vi "Package Measurement.vi"() -> ()   [LabVIEW 2021]
uses:
  _Measurement Packager Utility/Packager Helpers/Queue Driver/controls/Queue Operations.ctl
  <vilib>/Utility/miscctls.llb/LVRowAndColumnTypeDef.ctl
  _Measurement Packager Utility/Packager Helpers/controls/Config File Operations.ctl
  _Measurement Packager Utility/Packager Helpers/controls/Data Holder.ctl
  <vilib>/Utility/miscctls.llb/LVPoint32TypeDef.ctl
  _Measurement Packager Utility/Packager Helpers/controls/Build Spec Details.ctl
  <vilib>/AppBuilder/AB_API_Simple/Get Build Specification Version (path).vi
  _Measurement Packager Utility/Packager Helpers/Queue Driver/Queue Driver.lvlib
  _Measurement Packager Utility/Packager Helpers/Packager Helpers.lvlib
  _Measurement Packager Utility/Packager Helpers/Dictionary/Dictionary.lvlib
  <vilib>/AppBuilder/AB_API_Simple/NI_App_Builder_API.lvlib
panel:
  out "error out":errorcluster
  out "Tab Control":T1(tab)
  in  "Open Directory":bool
  in  "Feed Path":path
  out "Warning":bool=TRUE caption="Feed Path cannot be empty/invalid"
  in  "Next to select":bool
  in  "Build Package":bool
  in  "Project":path caption="LabVIEW Project Path"
  in  "Feed":T2(radio)
  in  "Back 1":bool
  in  "Populate Package":bool
  in  "Select All":bool
  out "Measurement List":i32(listbox)=-1 caption="Select the Measurements to build the package"
  out "Selection warning":string="Selected Project doesn't have EXE build spec"
  out "Maintainer Warning":string
  in  "Settings Page":enum32{"Page 1", "Page 2"}(tab)
  in  "Maintainer Email ID":string="sabthagiri@ni.com"
  in  "Architecture":string(combo)="1"
  in  "Maintainer":string="NI"
  in  "Back 2":bool
  in  "Start Build":bool
  in  "Package List":i32[](listbox) caption="Edit the Package Name and Version"
  in  "Settings":bool
  in  "Progres Bar":i32(slide)=9 caption="Creating Distribution..." scale=0.0..100.0
  in  "Start Next":bool
  in  "Log":bool[](array[boolean])=[TRUE, TRUE]
  in  "Build Status":i32(listbox)=-1
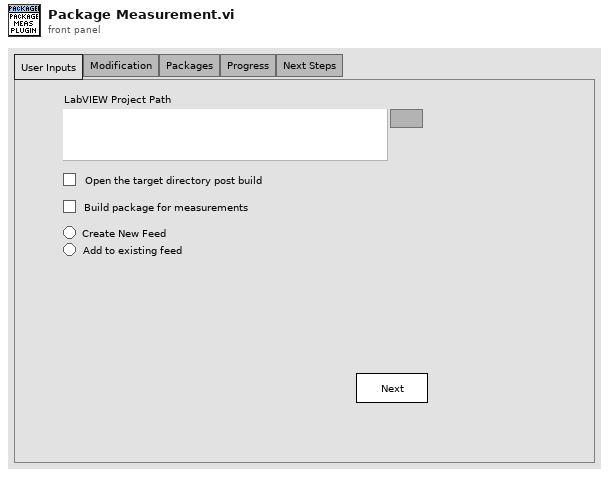
[diagram p1: front panel]
types:
  T1 = enum32{"User Inputs", "Modification", "Packages", "Progress", "Next Steps"}
  T2 = enum32{"No Selection", "CreateFeed", "AddtoFeed"}
  T3 = typedef "LVRowAndColumnTypeDef.ctl" = cluster{"Row":i32, "Column":i32}
  T4 = typedef "Queue Driver.lvlib/Queue Operations.ctl" = enum16{"Create Q", "Enqueue", "Enqueue N", "Dequeue", "Flush", "Release"}
  T5 = enum8{"Enabled", "Disabled", "Disabled and Grayed Out"}
  T6 = typedef "Packager Helpers.lvlib/Config File Operations.ctl" = enum16{"Read", "Write"}
  T7 = typedef "Packager Helpers.lvlib/Data Holder.ctl" = cluster{"Next Clicked?":bool, "MosueDown Coords":T8, "Build Spec":T9[], "No of Meas":i32, "No. of Selected Meas":i32, "Selected Meas":T9[], "Package Details":string[][], "Build Packge?":bool, "Packages Path":path, "Feed":enum32{"No Selection", "CreateFeed", "AddtoFeed"}, "Feed Path":path, "Valid Inputs?":bool, "Feed Old":enum32{"No Selection", "CreateFeed", "AddtoFeed"}, "Status":string[], "Open Directory?":bool}
  T8 = typedef "LVPoint32TypeDef.ctl" = cluster{"Horizontal":i32, "Vertical":i32}
  T9 = typedef "Packager Helpers.lvlib/Build Spec Details.ctl" = cluster{"EXE Name":string, "Target path":path, "Has PPL?":bool, "PPL Name":string}
  T10 = typedef "NI_App_Builder_API.lvlib/Build Specification Version.ctl" = cluster{"Major":u16, "Minor":u16, "Fix":u16, "Build":u16}
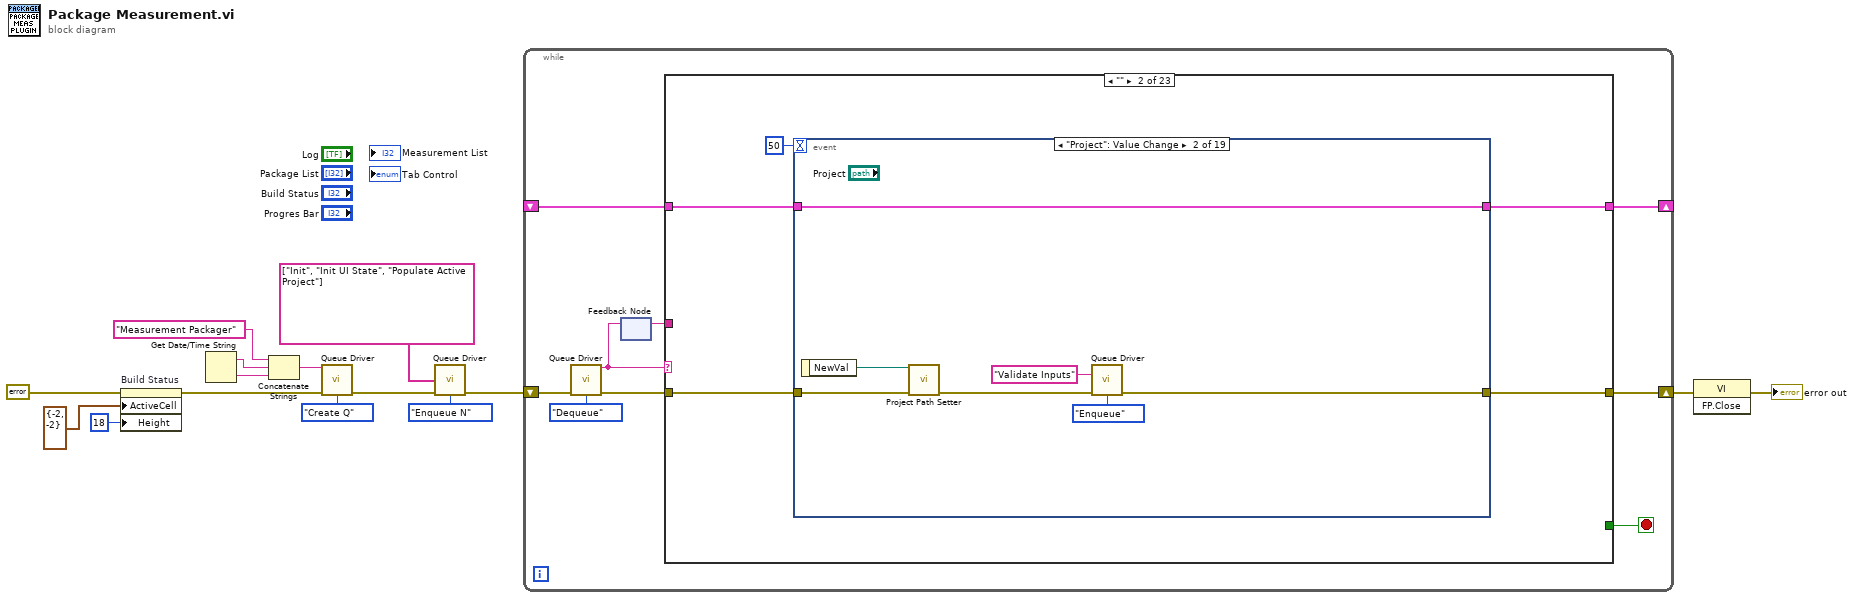
[diagram p0: block diagram]
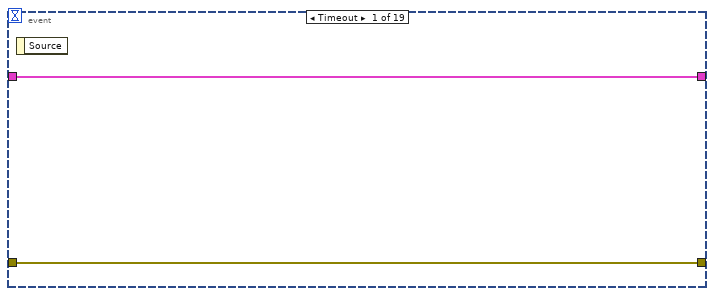
[diagram p3: hidden frame]
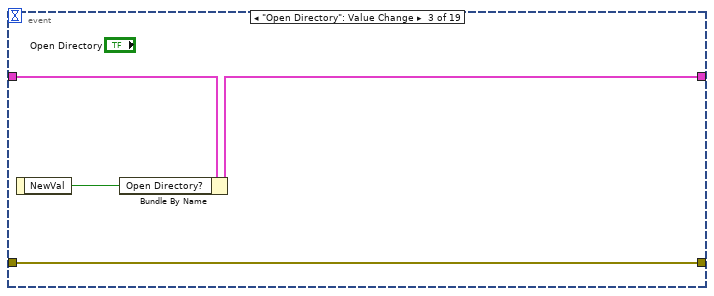
[diagram p4: hidden frame]
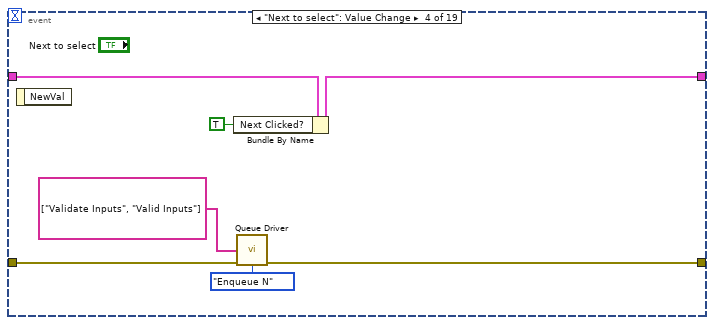
[diagram p5: hidden frame]
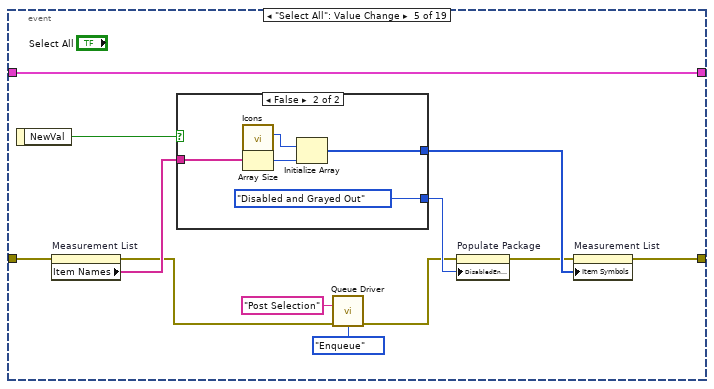
[diagram p6: hidden frame]
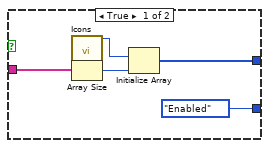
[diagram p7: hidden frame]
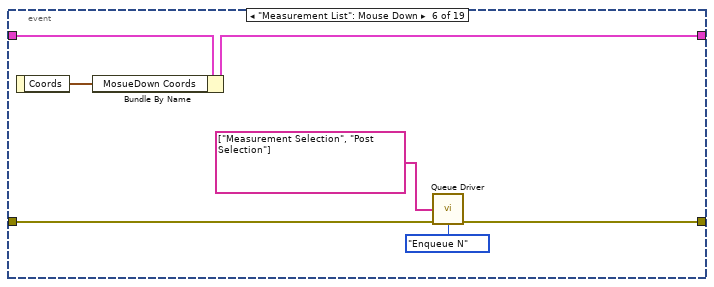
[diagram p8: hidden frame]
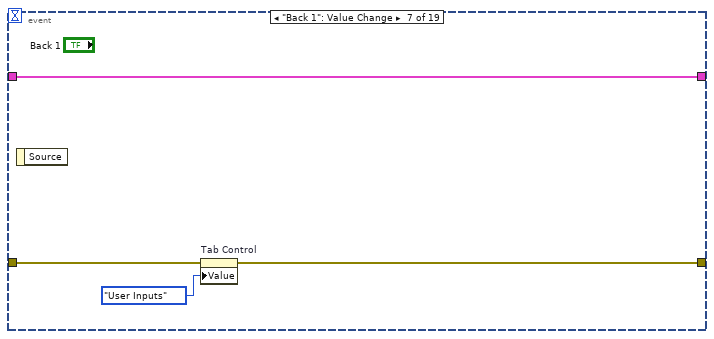
[diagram p9: hidden frame]
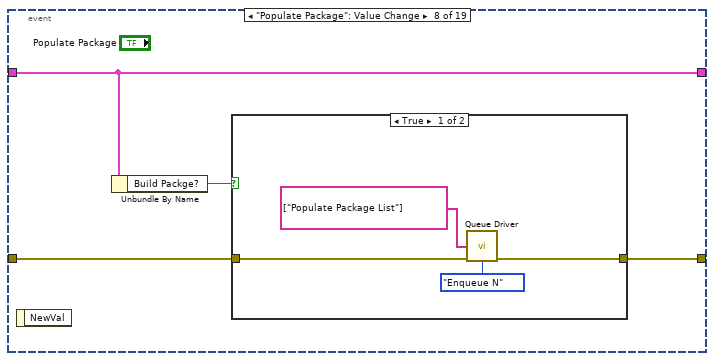
[diagram p10: hidden frame]
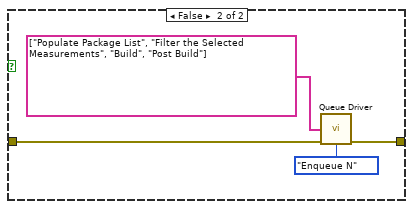
[diagram p11: hidden frame]
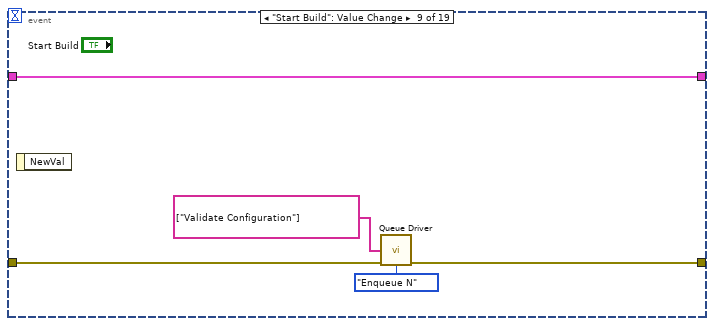
[diagram p12: hidden frame]
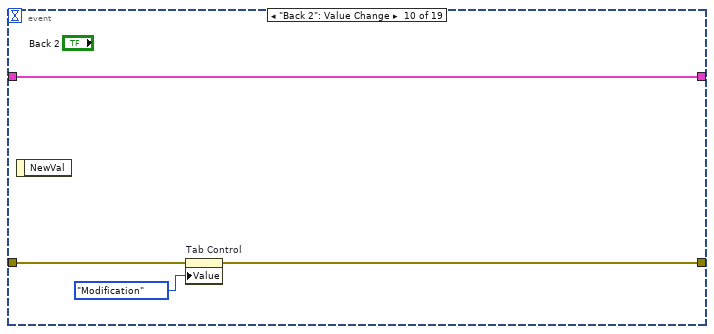
[diagram p13: hidden frame]
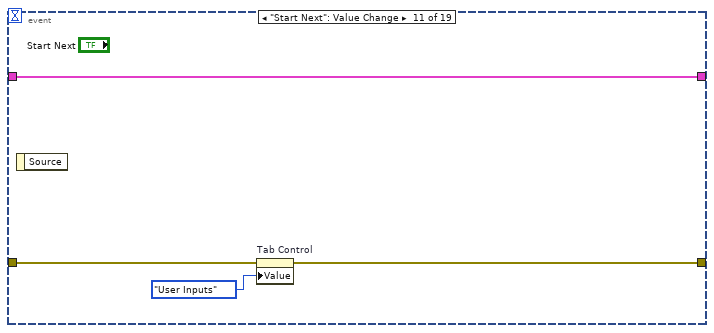
[diagram p14: hidden frame]
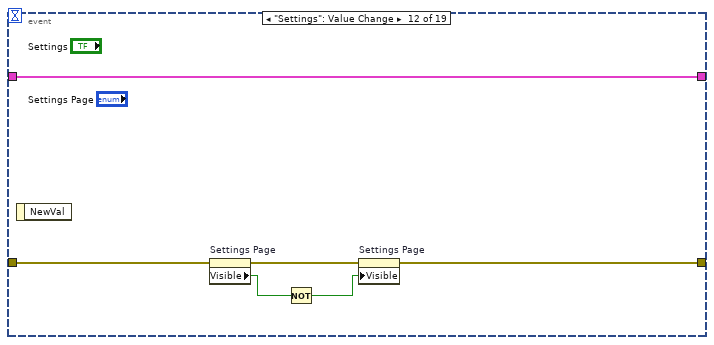
[diagram p15: hidden frame]
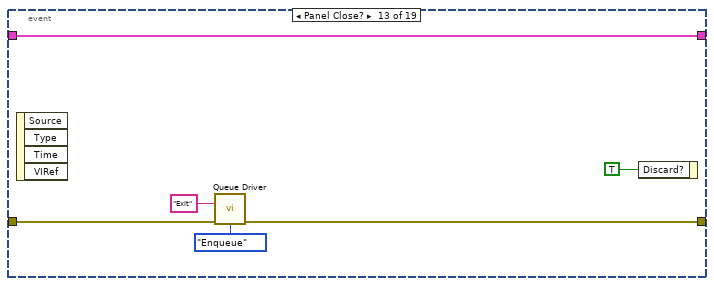
[diagram p16: hidden frame]
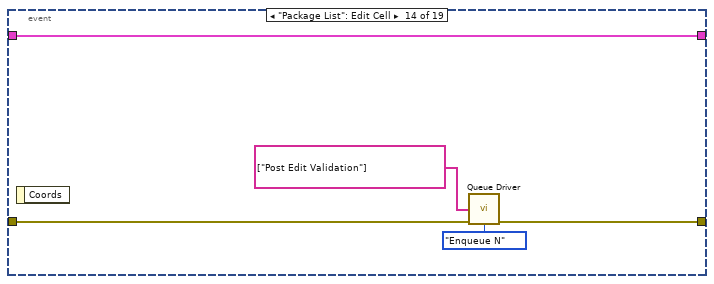
[diagram p17: hidden frame]
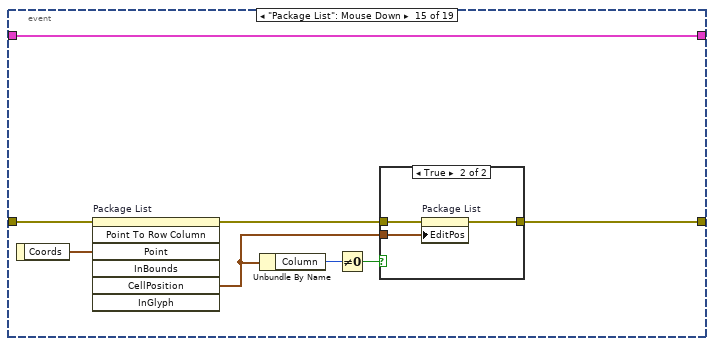
[diagram p18: hidden frame]
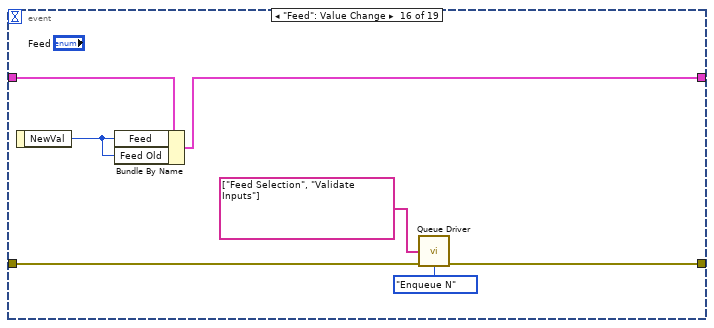
[diagram p20: hidden frame]
diagram:
  n1 = property on="Build Status" class="MCListbox (strict)"(error in=errorcluster {"status"=FALSE, "code"=0, "source"=""} ("error in (no error)"), "ActiveCell"=T3 {"Row"=-2, "Column"=-2} ("Active Cell:Active Cell"), "Height"=u32 18 ("Active Cell:Cell Size:Height")) -> (error out=w8:errorcluster)  [unwired: 1 in, 1 out]
  n2 = Get Date/Time String() -> (date string=w2:string, time string=w10:string)  [unwired: 3 in]
  n3 = Concatenate Strings("Measurement Packager" ("string"), w2, w10) -> (w9:string)
  n4 = call "Queue Driver.vi"("Name"=w9, "error in (no error)"=w8, "Queue Operations"=Queue_Operations."Create Q" ("Q Operations")) -> ("error out"=w13:errorcluster)  [unwired: 11 in, 1 out]
  n5 = call "Queue Driver.vi"("States[]"=string[] ["Init", "Init UI State", "Populate Active Project"], "error in (no error)"=w13, "Queue Operations"=Queue_Operations."Enqueue N" ("Q Operations")) -> ("error out"=w15:errorcluster)  [unwired: 11 in, 1 out]
  n6 = while {
    shift-right: [w17] -> w4
    shift-left: w15 -> [w24]
    shift-right: [w21] -> _
    shift-left: _ -> [w20]
    stop <- w18 stop-if-true
    n7 = call "Queue Driver.vi"("error in (no error)"=w24, "Queue Operations"=Queue_Operations."Dequeue" ("Q Operations")) -> ("Dequeued State"=w16:string, "error out"=w22:errorcluster)  [unwired: 12 in]
    n8 = feedback #1() -> (w19:string)  [unwired: 1 in]
    n9 = feedback-in #1(w16) -> ()
    n10 = case shown="\"\"" w16 {
      tunnel: w22 -> [w25 w31 w170 w182 w196 w217 w229 w283 w300 w320 w335 w358 w377 w391 w397 w418 w454 w458 w472 w486 w502 w515 w520]
      tunnel: [w25 w27 w168 w173 w190 w216 w233 w282 w303 w319 w332 w350 w378 w390 w394 w412 w453 w456 w469 w481 w500 w511 w522] -> w17
      tunnel: [w26 w30 w171 w186 w204 w218 w232 w281 w305 w321 w337 w360 w385 w393 w404 w421 w455 w459 w465 w499 w504 w518 w523] -> w21
      tunnel: w20 -> [w26 w29 _ w186 w205 w218 w231 w281 w297 w321 w337 w360 w386 w393 w404 w419 w455 w461 w465 w495 w504 w518 w523]
      tunnel: w19 -> [_ _ _ _ _ _ _ _ _ _ _ _ _ _ _ _ _ _ _ _ _ _ _]
      tunnel: [_ _ _ _ _ _ _ _ _ _ _ _ _ _ _ _ _ _ _ _ _ _ TRUE] -> w18
      frame Default {
      }
      frame "" {
        n11 = event shown="[1] \"Project\": Value Change" {
          selector: _ -> [_ _ _ _ _ _ _ _ _ _ _ _ _ _ _ _ _ _ _]
          dyn-events: _ -> [_ _ _ _ _ _ _ _ _ _ _ _ _ _ _ _ _ _ _]
          timeout: 50 -> [_ _ _ _ _ _ _ _ _ _ _ _ _ _ _ _ _ _ _]
          tunnel: [w32 w34 w41 w45 w52 w75 w81 w85 w97 w104 w108 w112 w116 w122 w128 w139 w147 w153 w160] -> w27
          tunnel: w31 -> [w32 w36 w41 w46 w56 w74 w82 w86 w98 w105 w109 w113 w117 w123 w127 w140 w146 w154 w161]
          tunnel: [w33 w39 w43 w49 w63 w79 w84 w88 w101 w103 w107 w110 w120 w126 w134 w144 w151 w159 w165] -> w30
          tunnel: w29 -> [w33 w39 w44 w50 w63 w80 w84 w88 w101 w103 w107 w110 w120 w126 w134 w145 w152 w159 w166]
          event Timeout {
            n12 = event-data() -> ()  [unwired: 1 in, 1 out]
          }
          event "Project": Value Change {
            n13 = event-data() -> ("NewVal"=w38:path)  [unwired: 1 in]
            n14 = call "Project Path Setter.vi"("ProjectPath In"=w38, "error in (no error)"=w36) -> ("error out"=w35:errorcluster)  [unwired: 13 in]
            n15 = call "Queue Driver.vi"("State"="Validate Inputs", "error in (no error)"=w35, "Queue Operations"=Queue_Operations."Enqueue" ("Q Operations")) -> ("error out"=w34:errorcluster)  [unwired: 11 in, 1 out]
          }
          event "Open Directory": Value Change {
            n16 = event-data() -> ("NewVal"=w42:bool)  [unwired: 1 in]
            n17 = Bundle By Name(cluster=w44, "Open Directory?"=w42) -> (w43:T7)
          }
          event "Next to select": Value Change {
            n18 = event-data() -> ()  [unwired: 1 in, 1 out]
            n19 = Bundle By Name(cluster=w50, "Next Clicked?"=TRUE) -> (w49:T7)
            n20 = call "Queue Driver.vi"("States[]"=string[] ["Validate Inputs", "Valid Inputs"], "error in (no error)"=w46, "Queue Operations"=Queue_Operations."Enqueue N" ("Q Operations")) -> ("error out"=w45:errorcluster)  [unwired: 11 in, 1 out]
          }
          event "Select All": Value Change {
            n21 = event-data() -> ("NewVal"=w58:bool)  [unwired: 1 in]
            n22 = property on="Measurement List" class="LstBox (strict)"(error in=w56) -> (error out=w55:errorcluster, "Item Names"=w62:string[])  [unwired: 1 in, 1 out]
            n23 = case shown="False" w58 {
              tunnel: w62 -> [w67 w72]
              tunnel: [w66 w71] -> w61
              tunnel: [T5."Enabled" ("Disabled") T5."Disabled and Grayed Out" ("Disabled")] -> w60
              frame True {
                n24 = call "Icons.vi"() -> ("Selected"=w64:i32)  [unwired: 14 in, 1 out]
                n25 = Array Size(array=w67) -> (size(s)=w68:i32)
                n26 = Initialize Array(w64, w68) -> (w66:i32[])
              }
              frame False {
                n27 = call "Icons.vi"() -> ("Non Selected"=w70:i32)  [unwired: 14 in, 1 out]
                n28 = Array Size(array=w72) -> (size(s)=w73:i32)
                n29 = Initialize Array(w70, w73) -> (w71:i32[])
              }
            }
            n30 = call "Queue Driver.vi"("State"="Post Selection", "error in (no error)"=w55, "Queue Operations"=Queue_Operations."Enqueue" ("Q Operations")) -> ("error out"=w54:errorcluster)  [unwired: 11 in, 1 out]
            n31 = property on="Populate Package" class="Bool"(error in=w54, "DisabledEnum"=w60) -> (error out=w53:errorcluster)  [unwired: 1 in, 1 out]
            n32 = property on="Measurement List" class="LstBox (strict)"(error in=w53, "Item Symbols"=w61) -> (error out=w52:errorcluster)  [unwired: 1 in, 1 out]
          }
          event "Measurement List": Mouse Down {
            n33 = event-data() -> ("Coords"=w77:T8)  [unwired: 1 in]
            n34 = Bundle By Name(cluster=w80, "MosueDown Coords"=w77) -> (w79:T7)
            n35 = call "Queue Driver.vi"("States[]"=string[] ["Measurement Selection", "Post Selection"], "error in (no error)"=w74, "Queue Operations"=Queue_Operations."Enqueue N" ("Q Operations")) -> ("error out"=w75:errorcluster)  [unwired: 11 in, 1 out]
          }
          event "Back 1": Value Change {
            n36 = event-data() -> ()  [unwired: 1 in, 1 out]
            n37 = property on="Tab Control" class="TabCtl (strict)"(error in=w82, "Value"=T1."User Inputs" ("Tab Control")) -> (error out=w81:errorcluster)  [unwired: 1 in, 1 out]
          }
          event "Populate Package": Value Change {
            n38 = event-data() -> ()  [unwired: 1 in, 1 out]
            n39 = Unbundle By Name(w88) -> ("Build Packge?"=w87:bool)
            n40 = case shown="True" w87 {
              tunnel: w86 -> [w90 w94]
              tunnel: [w89 w93] -> w85
              frame True {
                n41 = call "Queue Driver.vi"("States[]"=string[] ["Populate Package List"], "error in (no error)"=w90, "Queue Operations"=Queue_Operations."Enqueue N" ("Q Operations")) -> ("error out"=w89:errorcluster)  [unwired: 11 in, 1 out]
              }
              frame False {
                n42 = call "Queue Driver.vi"("States[]"=string[] ["Populate Package List", "Filter the Selected Measurements", "Build", "Post Build"], "error in (no error)"=w94, "Queue Operations"=Queue_Operations."Enqueue N" ("Q Operations")) -> ("error out"=w93:errorcluster)  [unwired: 11 in, 1 out]
              }
            }
          }
          event "Start Build": Value Change {
            n43 = event-data() -> ()  [unwired: 1 in, 1 out]
            n44 = call "Queue Driver.vi"("States[]"=string[] ["Validate Configuration"], "error in (no error)"=w98, "Queue Operations"=Queue_Operations."Enqueue N" ("Q Operations")) -> ("error out"=w97:errorcluster)  [unwired: 11 in, 1 out]
          }
          event "Back 2": Value Change {
            n45 = event-data() -> ()  [unwired: 1 in, 1 out]
            n46 = property on="Tab Control" class="TabCtl (strict)"(error in=w105, "Value"=T1."Modification" ("Tab Control")) -> (error out=w104:errorcluster)  [unwired: 1 in, 1 out]
          }
          event "Start Next": Value Change {
            n47 = event-data() -> ()  [unwired: 1 in, 1 out]
            n48 = property on="Tab Control" class="TabCtl (strict)"(error in=w109, "Value"=T1."User Inputs" ("Tab Control")) -> (error out=w108:errorcluster)  [unwired: 1 in, 1 out]
          }
          event "Settings": Value Change {
            n49 = event-data() -> ()  [unwired: 1 in, 1 out]
            n50 = property on="Settings Page" class="TabCtl (strict)"(error in=w113) -> (error out=w111:errorcluster, "Visible"=w115:bool)  [unwired: 1 in, 1 out]
            n51 = Not(x=w115) -> (.not. x?=w114:bool)
            n52 = property on="Settings Page" class="TabCtl (strict)"(error in=w111, "Visible"=w114) -> (error out=w112:errorcluster)  [unwired: 1 in, 1 out]
          }
          event Panel Close? {
            n53 = event-data() -> ()  [unwired: 1 in, 4 out]
            n54 = call "Queue Driver.vi"("State"="Exit", "error in (no error)"=w117, "Queue Operations"=Queue_Operations."Enqueue" ("Q Operations")) -> ("error out"=w116:errorcluster)  [unwired: 11 in, 1 out]
            n55 = event-data("Discard?"=TRUE) -> ()  [unwired: 1 in, 1 out]
          }
          event "Package List": Edit Cell {
            n56 = event-data() -> ()  [unwired: 1 in, 1 out]
            n57 = call "Queue Driver.vi"("States[]"=string[] ["Post Edit Validation"], "error in (no error)"=w123, "Queue Operations"=Queue_Operations."Enqueue N" ("Q Operations")) -> ("error out"=w122:errorcluster)  [unwired: 11 in, 1 out]
          }
          event "Package List": Mouse Down {
            n58 = event-data() -> ("Coords"=w133:T8)  [unwired: 1 in]
            n59 = invoke on="Package List" class="MCListbox (strict)" method="Point To Row Column"(error in=w127, "Point"=w133) -> (error out=w129:errorcluster, "CellPosition"=w130:T3)  [unwired: 5 in, 5 out]
            n60 = Unbundle By Name(w130) -> ("Column"=w132:i32)
            n61 = Not Equal To 0?(x=w132) -> (x != 0?=w131:bool)
            n62 = case shown="True" w131 {
              tunnel: w130 -> [_ w138]
              tunnel: w129 -> [w135 w137]
              tunnel: [w135 w136] -> w128
              frame False {
              }
              frame True {
                n63 = property on="Package List" class="MCListbox (strict)"(error in=w137, "EditPos"=w138) -> (error out=w136:errorcluster)  [unwired: 1 in, 1 out]
              }
            }
          }
          event "Feed": Value Change {
            n64 = event-data() -> ("NewVal"=w141:T2)  [unwired: 1 in]
            n65 = Bundle By Name(cluster=w145, "Feed"=w141, "Feed Old"=w141) -> (w144:T7)
            n66 = call "Queue Driver.vi"("States[]"=string[] ["Feed Selection", "Validate Inputs"], "error in (no error)"=w140, "Queue Operations"=Queue_Operations."Enqueue N" ("Q Operations")) -> ("error out"=w139:errorcluster)  [unwired: 11 in, 1 out]
          }
          event "Build Package": Value Change {
            n67 = event-data() -> ("NewVal"=w148:bool)  [unwired: 1 in]
            n68 = Bundle By Name(cluster=w152, "Build Packge?"=w148) -> (w151:T7)
            n69 = call "Queue Driver.vi"("States[]"=string[] ["Build Package Value Change", "Validate Inputs"], "error in (no error)"=w146, "Queue Operations"=Queue_Operations."Enqueue N" ("Q Operations")) -> ("error out"=w147:errorcluster)  [unwired: 11 in, 1 out]
          }
          event "Architecture", "Maintainer", "Maintainer Email ID": Value Change {
            n70 = event-data() -> ()  [unwired: 1 in, 1 out]
            n71 = call "Read or Write Configurations.vi"("Architecture"="Architecture", "Maintainer"="Maintainer", "Email"="Maintainer Email ID", "error in (no error)"=w154, "Operation"=Config_File_Operations."Write") -> ("error out"=w153:errorcluster)  [unwired: 7 in, 3 out]
          }
          event "Feed Path": Value Change {
            n72 = event-data() -> ("NewVal"=w162:path)  [unwired: 1 in]
            n73 = Bundle By Name(cluster=w166, "Feed Path"=w162) -> (w165:T7)
            n74 = call "Queue Driver.vi"("States[]"=string[] ["Validate Inputs"], "error in (no error)"=w161, "Queue Operations"=Queue_Operations."Enqueue N" ("Q Operations")) -> ("error out"=w160:errorcluster)  [unwired: 11 in, 1 out]
          }
        }
      }
      frame "Init" {
        w167 = TRUE ("Open Directory?")
        n75 = invoke class="VI" method="Default Vals.Reinit All"(error in=w170) -> (error out=w169:errorcluster)  [unwired: 2 in, 2 out]
        n76 = property on="Open Directory" class="Bool (strict)"(error in=w169, "Value"=w167) -> (error out=w168:errorcluster)  [unwired: 1 in, 1 out]
        n77 = Bundle By Name(cluster=T7 {"Next Clicked?"=TRUE, "MosueDown Coords"={"Horizontal"=0, "Vertical"=0}, "Build Spec"=[], "No of Meas"=0, "No. of Selected Meas"=0, "Selected Meas"=[], "Package Details"=[], "Build Packge?"=FALSE, "Packages Path"=path "", "Feed"=enum."No Selection", "Feed Path"=path "", "Valid Inputs?"=FALSE, "Feed Old"=enum."No Selection", "Status"=[], "Open Directory?"=FALSE}, "Open Directory?"=w167) -> (w171:T7)
      }
      frame "Init UI State" {
        w183 = u32 16448250 ("Selection Color")
        w184 = FALSE ("Visible")
        n78 = property on="Tab Control" class="TabCtl (strict)"(error in=w182, "Value"=T1."User Inputs" ("Tab Control")) -> (error out=w181:errorcluster)  [unwired: 1 in, 1 out]
        n79 = property on="Settings Page" class="TabCtl (strict)"(error in=w181, "Visible"=w184) -> (error out=w180:errorcluster)  [unwired: 1 in, 1 out]
        n80 = property on="Warning" class="Bool"(error in=w180, "Visible"=w184) -> (error out=w179:errorcluster)  [unwired: 1 in, 1 out]
        n81 = property on="Selection warning" class="Str"(error in=w179, "Visible"=w184) -> (error out=w178:errorcluster)  [unwired: 1 in, 1 out]
        n82 = property on="Feed Path" class="Path"(error in=w178, "Visible"=w184) -> (error out=w177:errorcluster)  [unwired: 1 in, 1 out]
        n83 = property on="Settings" class="Bool"(error in=w177, "Visible"=w184) -> (error out=w176:errorcluster)  [unwired: 1 in, 1 out]
        n84 = property on="Measurement List" class="LstBox (strict)"(error in=w176, "SelColor"=w183) -> (error out=w175:errorcluster)  [unwired: 1 in, 1 out]
        n85 = property on="Package List" class="MCListbox (strict)"(error in=w175, "SelColor"=w183) -> (error out=w174:errorcluster)  [unwired: 1 in, 1 out]
        n86 = property on="Build Status" class="MCListbox (strict)"(error in=w174, "SelColor"=w183) -> (error out=w173:errorcluster)  [unwired: 1 in, 1 out]
        "Selection warning" <- "Atleast one measurement should be selected" ("Selection warning")
        "Maintainer Warning" <- "Maintainer and Email ID cannot be empty" ("Maintainer Warning")
        "Warning" <- TRUE ("Warning")
      }
      frame "Populate Active Project" {
        # "Get the active labview project"
        n87 = call "Get Active ProjectPath.vi"("error in (no error)"=w196) -> ("Project Path"=w197:path, "error out"=w195:errorcluster)  [unwired: 13 in]
        n88 = property on="Project" class="Path"(error in=w195, "Value"=w197) -> (error out=w194:errorcluster)  [unwired: 1 in, 1 out]
        n89 = call "Project Path Setter.vi"("ProjectPath In"=w197, "error in (no error)"=w194) -> ("error out"=w193:errorcluster)  [unwired: 13 in]
        n90 = Empty String/Path?(string/path=w197) -> (empty?=w200:bool)
        n91 = Not A Number/Path/Refnum?(number/path/refnum=w197) -> (NaN/Path/Refnum?=w199:bool)
        n92 = Or(x=w199, y=w200) -> (x .or. y?=w198:bool)
        n93 = case "Not a valid path?" shown="False" w198 {
          tunnel: w205 -> [w210 w215]
          tunnel: [w209 w214] -> w204
          tunnel: [w207 w213] -> w203
          tunnel: [T5."Disabled and Grayed Out" ("Disabled") T5."Enabled" ("Disabled")] -> w201
          frame True {
            w207 = T2."No Selection" ("Feed")
            n94 = Bundle By Name(cluster=w210, "Build Packge?"=FALSE, "Feed"=w207) -> (w209:T7)
          }
          frame False {
            w213 = T2."CreateFeed" ("Feed")
            n95 = Bundle By Name(cluster=w215, "Build Packge?"=TRUE, "Feed"=w213) -> (w214:T7)
          }
        }
        n96 = Not(x=w198) -> (.not. x?=w202:bool)
        n97 = property on="Build Package" class="Bool (strict)"(error in=w193, "Value"=w202) -> (error out=w192:errorcluster)  [unwired: 1 in, 1 out]
        n98 = property on="Feed" class="RadioBtnsControl (strict)"(error in=w192, "DisabledEnum"=w201) -> (error out=w191:errorcluster)  [unwired: 1 in, 1 out]
        n99 = property on="Feed" class="RadioBtnsControl (strict)"(error in=w191, "Value"=w203) -> (error out=w190:errorcluster)  [unwired: 1 in, 1 out]
      }
      frame "Populate Config" {
        # "Disabling it because the config will not be populated in UI"
        # "Populate Config Data"
        n100 = disable-structure shown="Disabled" {
          disable-tunnel: w217 -> [w223 w228]
          disable-tunnel: [w219 w228] -> w216
          frame Disabled {
            n101 = call "Read or Write Configurations.vi"("error in (no error)"=w223, "Operation"=Config_File_Operations."Read") -> ("Architecture Out"=w226:string, "Maintainer Out"=w225:string, "Email Out"=w224:string, "error out"=w222:errorcluster)  [unwired: 10 in]
            n102 = property on="Maintainer Email ID" class="Str"(error in=w222, "Value"=w224) -> (error out=w221:errorcluster)  [unwired: 1 in, 1 out]
            n103 = property on="Maintainer" class="Str"(error in=w221, "Value"=w225) -> (error out=w220:errorcluster)  [unwired: 1 in, 1 out]
            n104 = property on="Architecture" class="CmbBox"(error in=w220, "Value"=w226) -> (error out=w219:errorcluster)  [unwired: 1 in, 1 out]
          }
          frame Enabled {
          }
        }
      }
      frame "Validate Inputs" {
        # "Validate Inputs"
        n105 = call "Validate Project Path.vi"("error in (no error)"=w229) -> ("Valid Path?"=w230:bool, "error out"=w234:errorcluster)  [unwired: 13 in]
        n106 = case "Valid project?" shown="True" w230 {
          tunnel: w234 -> [w241 w243]
          tunnel: [w240 w244] -> w233
          tunnel: [w238 w245] -> w232
          tunnel: w231 -> [w239 w246]
          frame False {
            n107 = property on="Warning" class="Bool"(error in=w241, "Visible"=TRUE, "Caption.Text"="Existing LabVIEW Project Path should be selected" ("Boolean Text.Text")) -> (error out=w240:errorcluster)  [unwired: 1 in, 1 out]
            n108 = Bundle By Name(cluster=w239, "Valid Inputs?"=FALSE) -> (w238:T7)
          }
          frame True {
            n109 = Unbundle By Name(w246) -> ("Build Packge?"=w242:bool, "Feed"=w248:T2, "Feed Path"=w247:path)
            n110 = case "Build package ?" shown="True" w242 {
              tunnel: w243 -> [w250 w260]
              tunnel: w248 -> [_ w259]
              tunnel: w247 -> [_ w258]
              tunnel: w246 -> [w254 w257]
              tunnel: [w253 w256] -> w245
              tunnel: [w249 w255] -> w244
              frame False {
                # "Invalid project Path"
                n111 = Bundle By Name(cluster=w254, "Valid Inputs?"=TRUE) -> (w253:T7)
                n112 = property on="Warning" class="Bool"(error in=w250, "Visible"=FALSE) -> (error out=w249:errorcluster)  [unwired: 1 in, 1 out]
              }
              frame True {
                n113 = case shown="\"AddtoFeed\"" w259 {
                  tunnel: w260 -> [w268 w274]
                  tunnel: w258 -> [w269 _]
                  tunnel: w257 -> [w273 w279]
                  tunnel: [w272 w278] -> w256
                  tunnel: [w271 w275] -> w255
                  frame "AddtoFeed" {
                    # "Validate Path"
                    n114 = Empty String/Path?(string/path=w269) -> (empty?=w267:bool)
                    n115 = Not A Number/Path/Refnum?(number/path/refnum=w269) -> (NaN/Path/Refnum?=w266:bool)
                    n116 = call <vilib>:"Check if File or Folder Exists.vi"("error in (no error)"=w268, "path"=w269) -> ("error out"=w264:errorcluster, "file or folder exists?"=w265:bool)  [unwired: 7 in, 1 out]
                    n117 = Not(x=w265) -> (.not. x?=w263:bool)
                    n118 = Compound Arithmetic op=OR(w267, w266, w263) -> (w262:bool)
                    n119 = Not(x=w262) -> (.not. x?=w270:bool)
                    n120 = Bundle By Name(cluster=w273, "Valid Inputs?"=w270) -> (w272:T7)
                    n121 = property on="Warning" class="Bool"(error in=w264, "Visible"=w262, "Caption.Text"="Feed Path cannot be empty/invalid" ("Boolean Text.Text")) -> (error out=w271:errorcluster)  [unwired: 1 in, 1 out]
                  }
                  frame Default {
                    n122 = property on="Warning" class="Bool"(error in=w274, "Visible"=FALSE) -> (error out=w275:errorcluster)  [unwired: 1 in, 1 out]
                    n123 = Bundle By Name(cluster=w279, "Valid Inputs?"=TRUE) -> (w278:T7)
                  }
                }
              }
            }
          }
        }
      }
      frame "Valid Inputs" {
        # "Check if valid inputs and if next is clicked"
        n124 = Unbundle By Name(w281) -> ("Valid Inputs?"=w280:bool)
        n125 = case "Valid Inputs?" shown="True" w280 {
          tunnel: w283 -> [w284 w290]
          tunnel: [w284 w287] -> w282
          tunnel: w281 -> [_ w286]
          frame False {
          }
          frame True {
            n126 = Unbundle By Name(w286) -> ("Next Clicked?"=w285:bool)
            n127 = property on="Warning" class="Bool"(error in=w290, "Visible"=FALSE) -> (error out=w288:errorcluster)  [unwired: 1 in, 1 out]
            n128 = case "Next Clicked?" shown="True" w285 {
              tunnel: w288 -> [w291 w294]
              tunnel: [w291 w292] -> w287
              frame False {
              }
              frame True {
                n129 = call "Queue Driver.vi"("States[]"=string[] ["Populate Measurements", "Update Tab", "Validate Measurement"], "error in (no error)"=w294, "Queue Operations"=Queue_Operations."Enqueue N" ("Q Operations")) -> ("error out"=w292:errorcluster)  [unwired: 11 in, 1 out]
              }
            }
          }
        }
      }
      frame "Build Package Value Change" {
        # "Build Package Value Change Handling"
        n130 = Unbundle By Name(w297) -> ("Feed"=w299:T2, "Build Packge?"=w306:bool, "Feed Old"=w302:T2)
        n131 = case shown="True" w306 {
          tunnel: w297 -> [w310 w316]
          tunnel: [w309 w313] -> w305
          tunnel: [T5."Disabled and Grayed Out" ("Disabled") T5."Enabled" ("Disabled")] -> w296
          tunnel: w302 -> [w307 w312]
          tunnel: [_ w314] -> w301
          tunnel: w299 -> [w308 _]
          tunnel: [w307 w312] -> w298
          frame False {
            n132 = Bundle By Name(cluster=w310, "Feed Old"=w308) -> (w309:T7)
          }
          frame True {
            n133 = case shown="\"AddtoFeed\"" w312 {
              tunnel: [TRUE _] -> w314
              frame "AddtoFeed" {
              }
              frame Default {
              }
            }
            n134 = Bundle By Name(cluster=w316, "Feed"=w312) -> (w313:T7)
          }
        }
        n135 = property on="Feed Path" class="Path"(error in=w300, "Visible"=w301) -> (error out=w304:errorcluster)  [unwired: 1 in, 1 out]
        n136 = property on="Feed" class="RadioBtnsControl (strict)"(error in=w304, "DisabledEnum"=w296, "Value"=w298) -> (error out=w303:errorcluster)  [unwired: 1 in, 1 out]
      }
      frame "Feed Selection" {
        # "Feed Selection Value Change Handling"
        n137 = Unbundle By Name(w321) -> ("Feed"=w318:T2)
        n138 = case shown="\"AddtoFeed\"" w318 {
          tunnel: w320 -> [w324 w327]
          tunnel: [w323 w326] -> w319
          frame Default {
            n139 = property on="Feed Path" class="Path"(error in=w324, "Visible"=FALSE) -> (error out=w323:errorcluster)  [unwired: 1 in, 1 out]
          }
          frame "AddtoFeed" {
            n140 = property on="Feed Path" class="Path"(error in=w327, "Visible"=TRUE) -> (error out=w326:errorcluster)  [unwired: 1 in, 1 out]
          }
        }
      }
      frame "Measurement Selection" {
        # "Measurement Selection Value change"
        n141 = Unbundle By Name(w337) -> ("No of Meas"=w329:i32, "MosueDown Coords"=w328:T8)
        n142 = property on="Measurement List" class="LstBox (strict)"(error in=w335) -> (error out=w334:errorcluster, "Item Symbols"=w336:i32[])  [unwired: 1 in, 1 out]
        n143 = invoke on="Measurement List" class="LstBox (strict)" method="Point To Row"(error in=w334, "Point"=w328) -> (error out=w333:errorcluster, "Row"=w331:i32)  [unwired: 5 in, 5 out]
        n144 = Greater?(x=w329, y=w331) -> (0:w330:bool)
        n145 = case "Mouse click In range?" shown="True" w330 {
          tunnel: w336 -> [_ w343]
          tunnel: w331 -> [_ w342]
          tunnel: w333 -> [w338 w340]
          tunnel: [w338 w339] -> w332
          frame False {
          }
          frame True {
            # "Change the item symbols"
            n146 = in-place {
              n147 = in-place-array #2(w343, w342) -> (w347:i32)
              n148 = call "Icons.vi"() -> ("Selected"=w344:i32, "Non Selected"=w348:i32)  [unwired: 14 in]
              n149 = Equal?(x=w347, y=w344) -> (x = y?=w346:bool)
              n150 = Swap Values(12:w344, 13:w346, 14:w348) -> (1:w345:i32)  [unwired: 1 out]
              n151 = in-place-array #2(w345) -> (w341:i32[])  [unwired: 1 out]
            }
            n152 = property on="Measurement List" class="LstBox (strict)"(error in=w340, "Item Symbols"=w341) -> (error out=w339:errorcluster)  [unwired: 1 in, 1 out]
          }
        }
      }
      frame "Post Selection" {
        # "Selection change handling"
        n153 = property on="Measurement List" class="LstBox (strict)"(error in=w358) -> (error out=w357:errorcluster, "Item Symbols"=w359:i32[])  [unwired: 1 in, 1 out]
        n154 = call "Check the Symbols.vi"("Item Symbols"=w359) -> ("All Selected?"=w349:bool, "None Selected"=w354:bool)  [unwired: 13 in]
        n155 = case "All selected?" shown="False" w349 {
          tunnel: [w366 T5."Enabled" ("Disabled")] -> w353
          tunnel: w357 -> [w363 w376]
          tunnel: [w365 w374] -> w356
          tunnel: w354 -> [w364 _]
          tunnel: [w361 _] -> w352
          frame False {
            n156 = property on="Select All" class="Bool (strict)"(error in=w363, "Value"=FALSE ("All")) -> (error out=w362:errorcluster)  [unwired: 1 in, 1 out]
            n157 = case "None Selected?" shown="True" w364 {
              tunnel: [T5."Enabled" ("Disabled") T5."Disabled and Grayed Out" ("Disabled")] -> w366
              tunnel: [w368 w371] -> w365
              tunnel: w362 -> [w368 w371]
              tunnel: [_ TRUE] -> w361
              frame False {
              }
              frame True {
              }
            }
          }
          frame True {
            n158 = property on="Select All" class="Bool (strict)"(error in=w376, "Value"=TRUE ("All")) -> (error out=w374:errorcluster)  [unwired: 1 in, 1 out]
          }
        }
        n159 = property on="Populate Package" class="Bool"(error in=w356, "DisabledEnum"=w353) -> (error out=w355:errorcluster)  [unwired: 1 in, 1 out]
        n160 = property on="Selection warning" class="Str"(error in=w355, "Visible"=w352, "Value"="Atleast one measurement should be selected" ("Selection warning")) -> (error out=w350:errorcluster)  [unwired: 1 in, 1 out]
      }
      frame "Populate Measurements" {
        # "Populate the selected measurements with the package name"
        n161 = call "Get all Build Spec Details.vi"("error in (no error)"=w377) -> ("Build Spec Details"=w384:T9[], "error out"=w379:errorcluster)  [unwired: 13 in]
        n162 = for {
          tunnel: w384 -> [w389] mode=indexing
          tunnel: [w388] -> w382 mode=indexing
          tunnel: [w387] -> w381 mode=indexing
          n163 = Unbundle By Name(w389) -> ("EXE Name"=w388:string)
          n164 = call "Icons.vi"() -> ("Selected"=w387:i32)  [unwired: 14 in, 1 out]
        }
        n165 = Array Size(array=w382) -> (size(s)=w380:i32)
        n166 = Bundle By Name(cluster=w386, "Build Spec"=w384, "No of Meas"=w380, "No. of Selected Meas"=w380) -> (w385:T7)
        n167 = property on="Measurement List" class="LstBox (strict)"(error in=w379, "Item Names"=w382, "Item Symbols"=w381, "Active Row"=-1 ("Selection Mode")) -> (error out=w378:errorcluster)  [unwired: 1 in, 1 out]
      }
      frame "Update Tab" {
        n168 = property on="Tab Control" class="TabCtl (strict)"(error in=w391, "Value"=T1."Modification" ("Tab Control")) -> (error out=w390:errorcluster)  [unwired: 1 in, 1 out]
      }
      frame "Validate Measurement" {
        # "Validate measurements"
        n169 = Unbundle By Name(w404) -> ("Build Spec"=w399:T9[])
        n170 = Empty Array?(array=w399) -> (empty?=w398:bool)
        n171 = case shown="True" w398 {
          tunnel: [T5."Enabled" ("Disabled") T5."Disabled and Grayed Out" ("Disabled")] -> w403
          tunnel: [TRUE ("All") FALSE ("All")] -> w400
          frame False {
          }
          frame True {
          }
        }
        n172 = property on="Populate Package" class="Bool"(error in=w397, "DisabledEnum"=w403) -> (error out=w396:errorcluster)  [unwired: 1 in, 1 out]
        n173 = property on="Select All" class="Bool (strict)"(error in=w396, "Value"=w400, "DisabledEnum"=w403) -> (error out=w395:errorcluster)  [unwired: 1 in, 1 out]
        n174 = Not(x=w400) -> (.not. x?=w401:bool)
        n175 = property on="Selection warning" class="Str"(error in=w395, "Visible"=w401, "Value"="Selected Project doesn't have EXE build spec" ("Selection warning")) -> (error out=w394:errorcluster)  [unwired: 1 in, 1 out]
      }
      frame "Populate Package List" {
        # "Populate Package List"
        n176 = property on="Measurement List" class="LstBox (strict)"(error in=w418) -> (error out=w417:errorcluster, "Item Names"=w425:string[], "Item Symbols"=w424:i32[])  [unwired: 1 in, 1 out]
        n177 = call "Project Path Getter.vi"("error in (no error)"=w417) -> ("Path"=w409:path, "error out"=w416:errorcluster)  [unwired: 13 in]
        n178 = for {
          tunnel: w425 -> [w431] mode=indexing
          tunnel: w424 -> [w433] mode=indexing
          tunnel: [w431] -> w423 mode=indexing if=w430
          tunnel: [w432] -> w420 mode=indexing if=w430
          shift-right: [w427] -> w415
          shift-left: w416 -> [w428]
          tunnel: w409 -> [w426]
          n179 = call "Icons.vi"() -> ("Selected"=w429:i32)  [unwired: 14 in, 1 out]
          n180 = Equal?(x=w433, y=w429) -> (x = y?=w430:bool)
          n181 = case shown="True" w430 {
            tunnel: [_ w446] -> w432
            tunnel: w428 -> [w434 w438]
            tunnel: w431 -> [_ w447]
            tunnel: [w434 w436] -> w427
            tunnel: w426 -> [_ w435]
            frame False {
            }
            frame True {
              n182 = call-poly <vilib>:"Get Build Specification Version.vi"("error in (no error)"=w438, "Name of build specification"=w447, "Path to project"=w435) -> ("error out"=w437:errorcluster, "Build Specification Version"=w441:T10)  [unwired: 7 in]
              n183 = call "Check Initial Version.vi"("Build Version In"=w441) -> ("Build Version Out"=w440:T10)  [unwired: 14 in]
              n184 = Unbundle By Name(w440) -> ("Major"=w445:u16, "Minor"=w444:u16, "Fix"=w443:u16, "Build"=w442:u16)
              n185 = Format Into String(format string="%d.%d.%d.%d", error in=w437, w445, w444, w443, w442) -> (resulting string=w446:string, error out=w436:errorcluster)  [unwired: 1 in]
            }
          }
        }
        n186 = Build Array(w423, w420) -> (w411:string[][])
        n187 = Transpose 2D Array(2D array=w411) -> (transposed array=w414:string[][])
        n188 = property on="Package List" class="MCListbox (strict)"(error in=w415, "ItemNames"=w414, "SelMode"=0 ("Selection Mode")) -> (error out=w413:errorcluster)  [unwired: 1 in, 1 out]
        n189 = Bundle By Name(cluster=w419, "Package Details"=w414) -> (w421:T7)
        n190 = property on="Tab Control" class="TabCtl (strict)"(error in=w413, "Value"=T1."Packages" ("Tab Control")) -> (error out=w412:errorcluster)  [unwired: 1 in, 1 out]
      }
      frame "Validate Configuration" {
        w451 = FALSE ("Visible")
        # "Check if configuration maintainer, maintainer email ID is valid"
        n191 = call "Queue Driver.vi"("States[]"=string[] ["Filter the Selected Measurements", "Build", "Post Build"], "error in (no error)"=w454, "Queue Operations"=Queue_Operations."Enqueue N" ("Q Operations")) -> ("error out"=w452:errorcluster)  [unwired: 11 in, 1 out]
        n192 = property on="Settings Page" class="TabCtl (strict)"(error in=w452, "Visible"=w451) -> (error out=w450:errorcluster)  [unwired: 1 in, 1 out]
        n193 = property on="Maintainer Warning" class="Str"(error in=w450, "Visible"=w451) -> (error out=w453:errorcluster)  [unwired: 1 in, 1 out]
      }
      frame "Filter the Selected Measurements" {
        # "Get the selected measurements"
        n194 = property on="Measurement List" class="LstBox (strict)"(error in=w458) -> (error out=w457:errorcluster, "Item Names"=w463:string[], "Item Symbols"=w464:i32[])  [unwired: 1 in, 1 out]
        n195 = Unbundle By Name(w461) -> ("Build Spec"=w462:T9[])
        n196 = call "Get Selected Measurements Data.vi"("Build Spec Details"=w462, "Item Names"=w463, "Item Symbols"=w464, "error in (no error)"=w457) -> ("Selected Measurements"=w460:T9[], "error out"=w456:errorcluster)  [unwired: 10 in]
        n197 = Bundle By Name(cluster=w461, "Selected Meas"=w460) -> (w459:T7)
      }
      frame "Post Edit Validation" {
        # "After editing validate if the changes are valid"
        n198 = Unbundle By Name(w465) -> ("Package Details"=w480:string[][])
        n199 = property on="Package List" class="MCListbox (strict)"(error in=w472) -> (error out=w471:errorcluster, "ItemNames"=w467:string[][])  [unwired: 1 in, 1 out]
        n200 = Index Array(array=w467, index (col)=1 ("disabled index (col)")) -> (element=w473:string[])  [unwired: 1 in]
        n201 = Index Array(array=w480, index (col) #1=0 ("disabled index (col)"), index (col) #2=1 ("disabled index (col)")) -> (element #1=w477:string[], element #2=w474:string[])  [unwired: 2 in]
        n202 = call "Validate the version.vi"("Old Version"=w474, "New Version"=w473, "error in (no error)"=w471) -> ("Version Out"=w475:string[], "error out"=w470:errorcluster)  [unwired: 11 in]
        n203 = Build Array(w477, w475) -> (w476:string[][])
        n204 = Transpose 2D Array(2D array=w476) -> (transposed array=w468:string[][])
        n205 = property on="Package List" class="MCListbox (strict)"(error in=w470, "ItemNames"=w468) -> (error out=w469:errorcluster)  [unwired: 1 in, 1 out]
      }
      frame "Build" {
        # "Start build process"
        n206 = property on="Tab Control" class="TabCtl (strict)"(error in=w486, "Value"=T1."Progress" ("Tab Control")) -> (error out=w485:errorcluster)  [unwired: 1 in, 1 out]
        n207 = property on="Progres Bar" class="Slide (strict)"(error in=w485, "Value"=2 ("Progres Bar")) -> (error out=w484:errorcluster)  [unwired: 1 in, 1 out]
        n208 = Unbundle By Name(w495) -> ("Build Packge?"=w491:bool, "Open Directory?"=w490:bool, "Feed"=w489:T2, "Feed Path"=w488:path, "Selected Meas"=w487:T9[])
        n209 = property on="Package List" class="MCListbox (strict)"(error in=w484) -> (error out=w483:errorcluster, "ItemNames"=w494:string[][])  [unwired: 1 in, 1 out]
        n210 = control-ref of="Progres Bar"() -> (w492:refnum<vi>)
        n211 = call "Start Build.vi"("Open Directory?"=w490, "Build Package?"=w491, "Progres Bar"=w492, "Feed"=w489, "Feed Path"=w488, "Selected Measurements"=w487, "error in (no error)"=w483, "Package Spec"=w494) -> ("Status"=w493:string[], "error out"=w482:errorcluster)  [unwired: 6 in]
        n212 = Bundle By Name(cluster=w495, "Status"=w493) -> (w499:T7)
        n213 = property on="Tab Control" class="TabCtl (strict)"(error in=w482, "Value"=T1."Next Steps" ("Tab Control")) -> (error out=w481:errorcluster)  [unwired: 1 in, 1 out]
      }
      frame "Post Build" {
        # "Populate the results in post build"
        n214 = Unbundle By Name(w504) -> ("Selected Meas"=w503:T9[], "Status"=w506:string[])
        n215 = for {
          tunnel: w503 -> [w509] mode=indexing
          tunnel: [w508] -> w507 mode=indexing
          n216 = Unbundle By Name(w509) -> ("EXE Name"=w508:string)
        }
        n217 = Build Array(w507, w506) -> (w505:string[][])
        n218 = Transpose 2D Array(2D array=w505) -> (transposed array=w501:string[][])
        n219 = property on="Build Status" class="MCListbox (strict)"(error in=w502, "ItemNames"=w501) -> (error out=w500:errorcluster)  [unwired: 1 in, 1 out]
      }
      frame "Error" {
        n220 = call <vilib>:"Simple Error Handler.vi"("error in (no error)"=w515) -> ("error out"=w514:errorcluster)  [unwired: 4 in, 4 out]
        n221 = call <vilib>:"Clear Errors.vi"("error in (no error)"=w514) -> ("error out"=w513:errorcluster)  [unwired: 5 in, 1 out]
        n222 = call "Queue Driver.vi"("error in (no error)"=w513, "Queue Operations"=Queue_Operations."Flush" ("Q Operations")) -> ("error out"=w512:errorcluster)  [unwired: 12 in, 1 out]
        n223 = call "Queue Driver.vi"("State"="Exit", "error in (no error)"=w512, "Queue Operations"=Queue_Operations."Enqueue" ("Q Operations")) -> ("error out"=w511:errorcluster)  [unwired: 11 in, 1 out]
      }
      frame "Exit" {
        n224 = call "Queue Driver.vi"("error in (no error)"=w520, "Queue Operations"=Queue_Operations."Flush" ("Q Operations")) -> ("error out"=w521:errorcluster)  [unwired: 12 in, 1 out]
        n225 = call "Queue Driver.vi"("error in (no error)"=w521, "Queue Operations"=Queue_Operations."Release" ("Q Operations")) -> ("error out"=w522:errorcluster)  [unwired: 12 in, 1 out]
      }
    }
  }
  n226 = invoke class="VI" method="FP.Close"(error in=w4) -> (error out=→"error out":errorcluster)  [unwired: 2 in, 2 out]
